vi "DMD_write.vi"(8 "String":string="C:\\Users\\1TEM\\Documents\\MATLAB\\MASKS\\UP.bmp", 11 "reference out":refnum<k24>) -> (0 "error out":errorcluster)   [LabVIEW 2017]
panel:
  out "result string":string
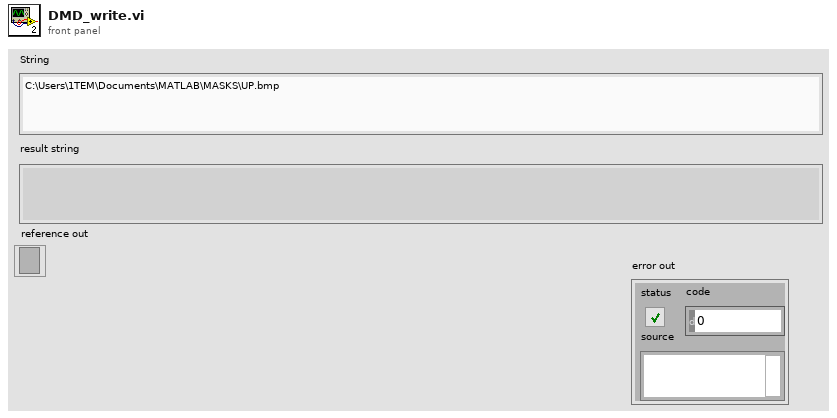
[diagram p1: front panel]
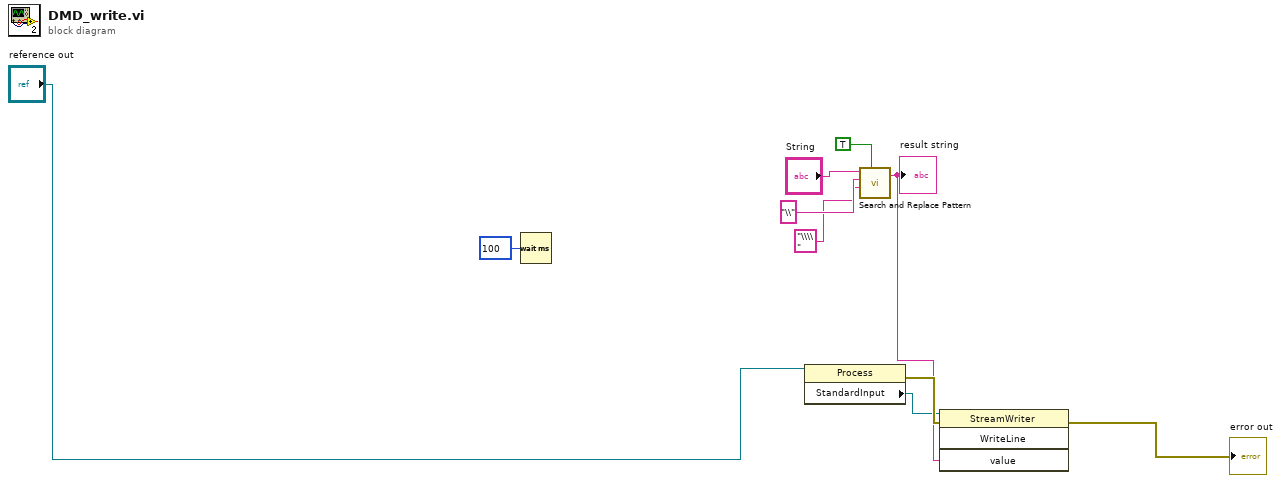
[diagram p0: block diagram]
diagram:
  n1 = Wait (ms)(milliseconds to wait=u32 100) -> ()  [unwired: 1 out]
  n2 = property class="Process"(reference="reference out") -> (error out=w10:errorcluster, "StandardInput"=w8:refnum<k24>)  [unwired: 1 in, 1 out]
  n3 = call <vilib>:"Search and Replace Pattern.vi"("string"="String", "regular expression (\"\")"="\\" ("regular expression (\"\")"), "replace string (\"\")"="\\\\" ("replace string (\"\")"), "replace all? (F)"=TRUE) -> ("result string"=w9:string)  [unwired: 1 in, 1 out]
  "result string" <- w9
  n4 = invoke class="StreamWriter" method="WriteLine"(reference=w8, error in=w10, "value"=w9) -> (error out=→"error out":errorcluster)  [unwired: 1 in, 3 out]
